vi "SPARK Get Limit Switch Config.vi"   [LabVIEW 2023]
doc: "Get the configuration of a limit switch connected to the data port of the SPARK."
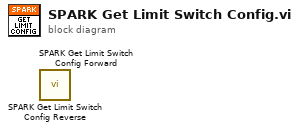
[diagram p0: block diagram]
diagram:
  n1 = call "SPARK Get Limit Switch Config Reverse.vi"() -> ()  [unwired: 8 in, 4 out]
  n2 = call "SPARK Get Limit Switch Config Forward.vi"() -> ()  [unwired: 8 in, 4 out]
